vi "Slam Loop.vi"() -> (3 "slam run time":u32)   [LabVIEW 2017]
uses:
  Control Globals.vi
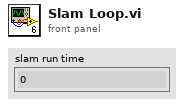
[diagram p1: front panel]
types:
  T1 = cluster{dbl[], dbl[], "Estimated Pose Delta":cluster{"X":dbl, "Y":dbl, "R":dbl}}
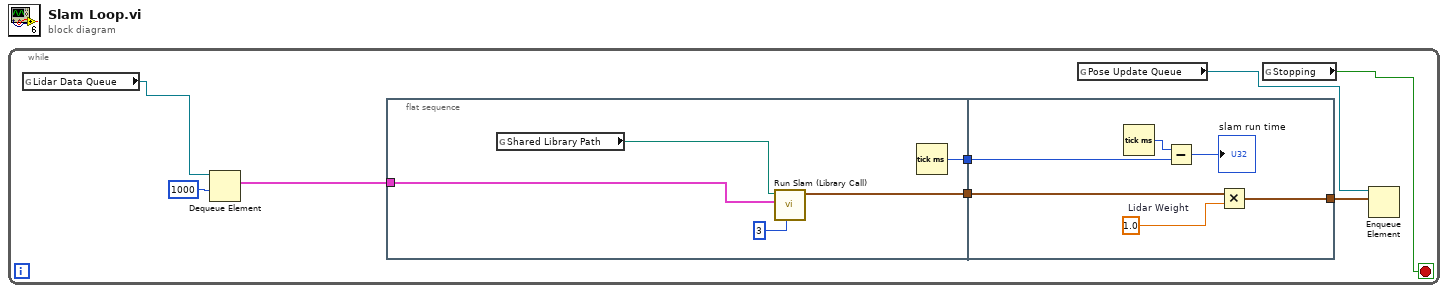
[diagram p0: block diagram]
diagram:
  n1 = while {
    stop <- w3 stop-if-true
    n2 = global read "Control Globals.vi" "Lidar Data Queue"() -> (w1:refnum<queue>)
    n3 = Dequeue Element(queue=w1, timeout in ms (-1)=1000) -> (element=w8:T1)  [unwired: 1 in, 3 out]
    n4 = flat-sequence {
      tunnel: w8 -> [w13]
      tunnel: [w12] -> w5
      tunnel: [w11] -> w4
      tunnel: [w16] -> w6
      tunnel: w5 -> [w14]
      tunnel: w4 -> [w19]
      frame #0 {
        n5 = global read "Control Globals.vi" "Shared Library Path"() -> (w9:path)
        n6 = call "Run Slam (Library Call).vi"("Itearations"=3, "Lidar Data"=w13, "Library Path"=w9) -> ("Pose Delta"=w12:cluster{"X":dbl, "Y":dbl, "R":dbl})  [unwired: 8 in]
        n7 = Tick Count (ms)() -> (millisecond timer value=w11:u32)
      }
      frame #1 {
        w15 = 1.0  # Lidar Weight
        n8 = Tick Count (ms)() -> (millisecond timer value=w18:u32)
        n9 = Subtract(x=w18, y=w19) -> (x-y=→"slam run time":u32)
        n10 = Multiply(x=w14, y=w15) -> (x*y=w16:cluster{"X":dbl, "Y":dbl, "R":dbl})
      }
    }
    n11 = global read "Control Globals.vi" "Pose Update Queue"() -> (w2:refnum<queue>)
    n12 = global read "Control Globals.vi" "Stopping"() -> (w3:bool)
    n13 = Enqueue Element(queue=w2, element=w6) -> ()  [unwired: 2 in, 3 out]
  }
